vi "show version of VIs.vi"() -> ()   [LabVIEW 2015]
panel:
  in  "Multicolumn Listbox":i32[](listbox)
  in  "folder path":path
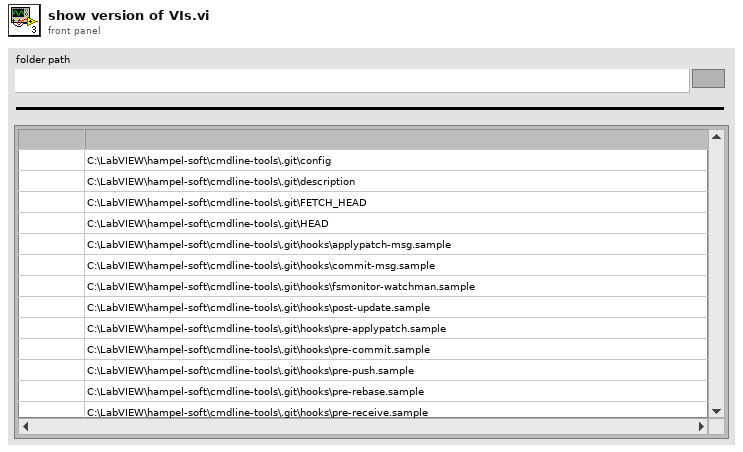
[diagram p1: front panel]
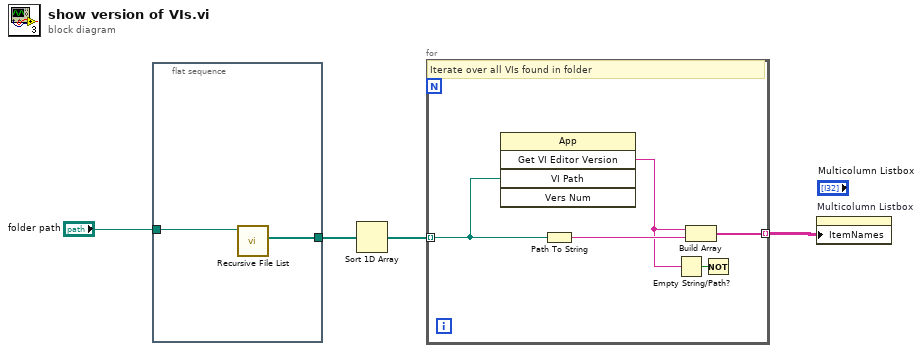
[diagram p0: block diagram]
diagram:
  n1 = flat-sequence {
    tunnel: "folder path" -> [w6]
    tunnel: [w5] -> w1
    frame #0 {
      n2 = call <vilib>:"Recursive File List.vi"("Folder Path"=w6) -> ("All Files in Dir"=w5:path[])  [unwired: 6 in, 4 out]
    }
  }
  n3 = Sort 1D Array(array=w1) -> (sorted array=w2:path[])
  n4 = for {
    tunnel: w2 -> [w11] mode=indexing
    tunnel: [w9] -> w3 mode=indexing
    # "Iterate over all VIs found in folder"
    n5 = invoke class="App" method="Get VI Editor Version"("VI Path"=w11) -> ("Get VI Editor Version"=w8:string)  [unwired: 4 in, 4 out]
    n6 = Path To String(path=w11) -> (string=w10:string)
    n7 = Empty String/Path?(string/path=w8) -> (empty?=w7:bool)
    n8 = Build Array(w8, w10) -> (w9:string[])
    n9 = Not(x=w7) -> ()  [unwired: 1 out]
  }
  n10 = property on="Multicolumn Listbox" class="MCListbox (strict)"("ItemNames"=w3) -> ()  [unwired: 2 in, 2 out]
